vi "Init.vi"(8 "error in (no error)":errorcluster, 11 "Coffee Actor in":refnum<class "Coffee Actor.lvclass">) -> (0 "error out":errorcluster, 3 "Coffee Actor out":refnum<class "Coffee Actor.lvclass">)   [LabVIEW 2020, in "Coffee Actor.lvlib" / "Coffee Actor.lvclass"]
uses:
  Coffee Actor.lvclass
  Coffee Actor.lvclass/Coffee Actor.ctl
  <vilib>/Utility/config.llb/Read Key (Double).vi
  <vilib>/Utility/config.llb/Read Key (String).vi
  <vilib>/Utility/config.llb/NI_LVConfig.lvlib
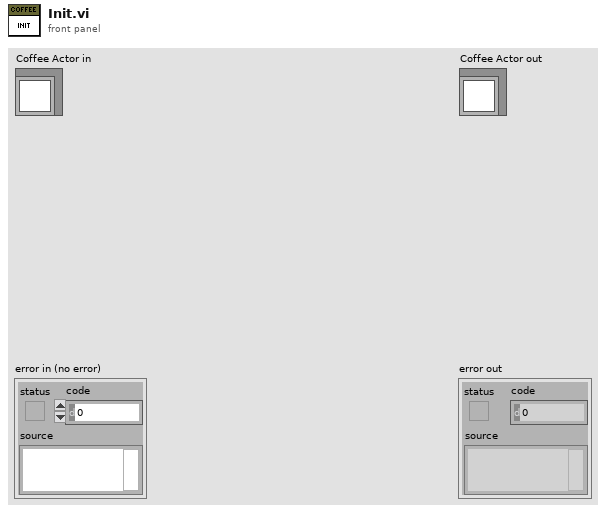
[diagram p1: front panel]
types:
  T1 = typedef "NI_LVConfig.lvlib/Config Data RefNum.ctl" = refnum<k1>
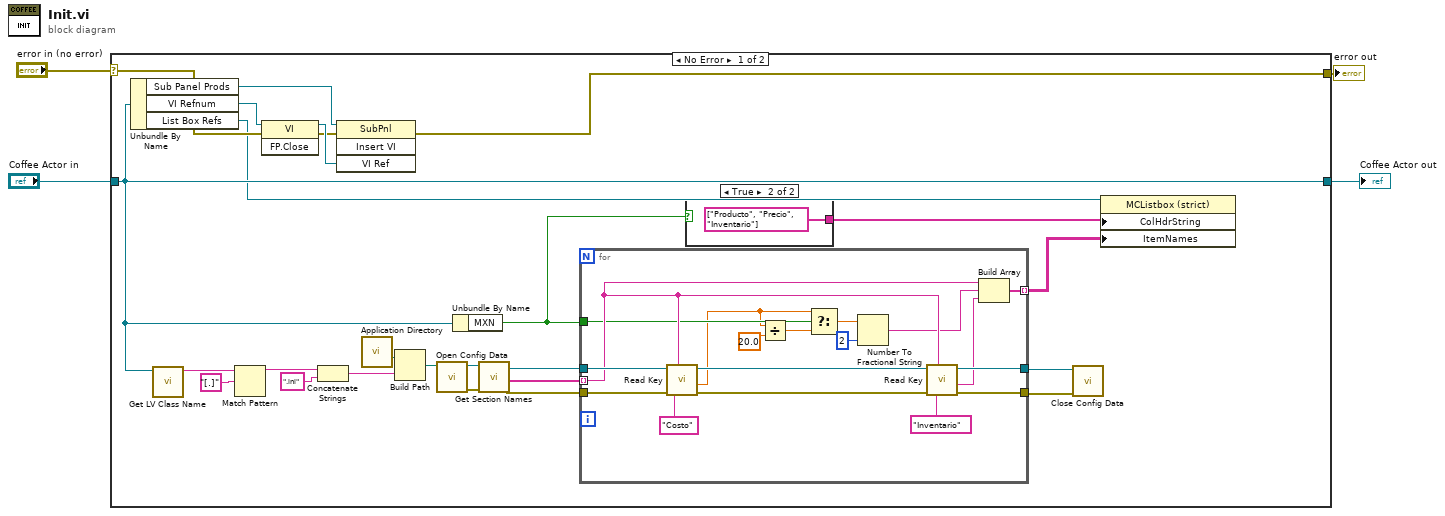
[diagram p0: block diagram]
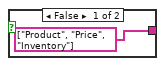
[diagram p2: hidden frame]
diagram:
  n1 = case shown="No Error" "error in (no error)" {
    selector: "error in (no error)" -> [w26 w51]
    tunnel: [w25 w51] -> w3
    tunnel: [w14 w50] -> w1
    tunnel: "Coffee Actor in" -> [w14 w50]
    frame No Error {
      n2 = Unbundle By Name(w14) -> ("Sub Panel Prods"=w24:refnum<vi>, "VI Refnum"=w27:refnum<vi>, "List Box Refs"=w8:refnum<vi>)
      n3 = call <vilib>:"Get LV Class Name.vi"("object"=w14) -> ("class name"=w18:string)  [unwired: 9 in, 1 out]
      n4 = Match Pattern(string=w18, regular expression="[.]") -> (before substring=w16:string)  [unwired: 1 in, 3 out]
      n5 = invoke class="VI" method="FP.Close"(reference=w27, error in=w26) -> (reference out=w29:refnum<vi>, error out=w28:errorcluster)  [unwired: 1 in, 1 out]
      n6 = Concatenate Strings(w16, ".ini" ("string")) -> (w21:string)
      n7 = invoke class="SubPnl" method="Insert VI"(reference=w24, error in=w28, "VI Ref"=w29) -> (error out=w25:errorcluster)  [unwired: 1 in, 3 out]
      n8 = call <vilib>:"Application Directory.vi"() -> ("Application Directory"=w23:path)
      n9 = Build Path(base path=w23, name or relative path=w21) -> (appended path=w20:path)
      n10 = call <vilib>:"Open Config Data.vi"("configuration file path"=w20) -> ("error out"=w19:errorcluster, "refnum"=w15:T1)  [unwired: 8 in, 1 out]
      n11 = Unbundle By Name(w14) -> ("MXN"=w5:bool)
      n12 = call <vilib>:"Get Section Names.vi"("error in (no error)"=w19, "refnum"=w15) -> ("error out"=w11:errorcluster, "section names"=w12:string[], "refnum out"=w13:T1)  [unwired: 7 in]
      n13 = for {
        tunnel: w13 -> [w49]
        tunnel: w11 -> [w48]
        tunnel: [w45] -> w9
        tunnel: [w44] -> w10
        tunnel: w5 -> [w36]
        tunnel: w12 -> [w42] mode=indexing
        tunnel: [w40] -> w6 mode=indexing
        n14 = call-poly <vilib>:"Read Key.vi"("section"=w42, "error in (no error)"=w48, "key"="Costo", "refnum"=w49) -> ("error out"=w47:errorcluster, "value"=w32:dbl, "refnum out"=w46:T1)  [unwired: 4 in, 1 out]
        n15 = Divide(x=w32, y=20.0) -> (x/y=w34:dbl)
        n16 = Select(t=w32, s=w36, f=w34) -> (s? t:f=w35:dbl)
        n17 = Number To Fractional String(number=w35, precision (6)=i16 2) -> (F-format string=w38:string)  [unwired: 2 in]
        n18 = call-poly <vilib>:"Read Key.vi"("section"=w42, "error in (no error)"=w47, "key"="Inventario", "refnum"=w46) -> ("error out"=w45:errorcluster, "value"=w41:string, "refnum out"=w44:T1)  [unwired: 4 in, 1 out]
        n19 = Build Array(w42, w38, w41) -> (w40:string[])
      }
      n20 = case shown="True" w5 {
        tunnel: [string[] ["Product", "Price", "Inventory"] ("Column Header Strings[]") string[] ["Producto", "Precio", "Inventario"] ("Column Header Strings[]")] -> w7
        frame False {
        }
        frame True {
        }
      }
      n21 = call <vilib>:"Close Config Data.vi"("error in (no error)"=w9, "refnum"=w10) -> ()  [unwired: 8 in, 2 out]
      n22 = property class="MCListbox (strict)"(reference=w8, "ColHdrString"=w7, "ItemNames"=w6) -> ()  [unwired: 1 in, 2 out]
    }
    frame Error {
    }
  }
  "error out" <- w3
  "Coffee Actor out" <- w1
